vi "sub_write_API_route_to_buf_file.vi"(8 "error in (no error)":errorcluster, 10 "API route":string, 11 "Buffer File in":refnum<file>) -> (0 "error out":errorcluster, 3 "Buffer File out":refnum<file>)   [LabVIEW 2013, in "daqio minimal.lvlib"]
doc: "This adds the API POST route as a header to a new buffer file."
uses:
  daqio minimal.lvlib
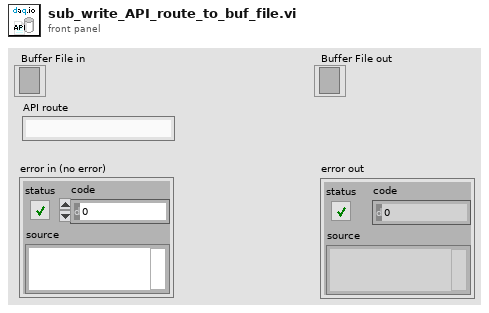
[diagram p1: front panel]
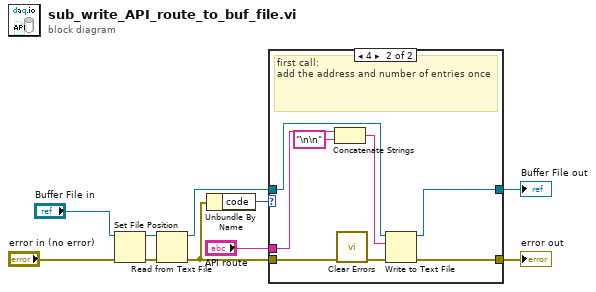
[diagram p0: block diagram]
diagram:
  n1 = Set File Position(refnum="Buffer File in", error in="error in (no error)") -> (refnum out=w6:refnum<file>, error out=w5:errorcluster)  [unwired: 2 in]
  n2 = Read from Text File(file (use dialog)=w6, error in=w5) -> (refnum out=w10:refnum<file>, error out=w8:errorcluster)  [unwired: 2 in, 2 out]
  n3 = Unbundle By Name(w8) -> ("code"=w7:i32)
  n4 = case shown="4" w7 {
    tunnel: [w12 w20] -> w2
    tunnel: [w11 w19] -> w1
    tunnel: w8 -> [w12 w18]
    tunnel: "API route" -> [_ w15]
    tunnel: w10 -> [w11 w14]
    frame 0, Default {
    }
    frame 4 {
      # "first call: \nadd the address and number of entries once"
      n5 = Concatenate Strings(w15, "\n\n" ("string")) -> (w16:string)
      n6 = call <vilib>:"Clear Errors.vi"("error in (no error)"=w18) -> ("error out"=w17:errorcluster)  [unwired: 6 in]
      n7 = Write to Text File(file (use dialog)=w14, text=w16, error in=w17) -> (refnum out=w19:refnum<file>, error out=w20:errorcluster)  [unwired: 1 in, 1 out]
    }
  }
  "error out" <- w2
  "Buffer File out" <- w1
